vi "D2SParser - Public - Function - Parse File.vi"(8 "error in (no error)":errorcluster, 11 "DS2 File":path) -> (0 "error out":errorcluster, 3 "D2Character":refnum<class "D2Character.lvclass">)   [LabVIEW 2015, in "D2SParser.lvclass"]
uses:
  D2SParser.lvclass
  D2Character/D2Character.lvclass
  D2SParser.lvclass/D2SParser.ctl
  D2SParser - Public - Accessors - Get D2 Character.vi
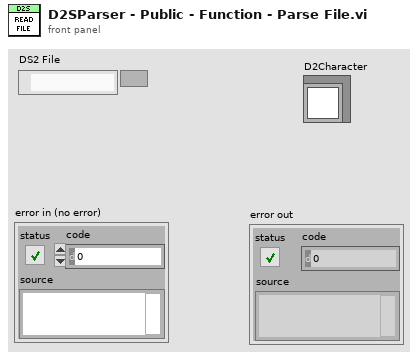
[diagram p1: front panel]
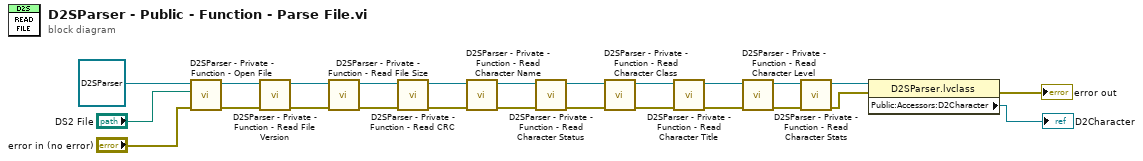
[diagram p0: block diagram]
diagram:
  n1 = call "D2SParser - Private - Function - Open File.vi"("error in (no error)"="error in (no error)", "Path"="DS2 File", "D2SParser in"=refnum<class "D2SParser.lvclass"> refnum) -> ("error out"=w15:errorcluster, "D2SParser out"=w22:refnum<class "D2SParser.lvclass">)  [unwired: 7 in]
  n2 = call "D2SParser - Private - Function - Read File Version.vi"("error in (no error)"=w15, "D2SParser in"=w22) -> ("error out"=w14:errorcluster, "D2SParser out"=w1:refnum<class "D2SParser.lvclass">)  [unwired: 8 in]
  n3 = call "D2SParser - Private - Function - Read File Size.vi"("error in (no error)"=w14, "D2SParser in"=w1) -> ("error out"=w13:errorcluster, "D2SParser out"=w21:refnum<class "D2SParser.lvclass">)  [unwired: 8 in]
  n4 = call "D2SParser - Private - Function - Read CRC.vi"("error in (no error)"=w13, "D2SParser in"=w21) -> ("error out"=w12:errorcluster, "D2SParser out"=w20:refnum<class "D2SParser.lvclass">)  [unwired: 8 in]
  n5 = call "D2SParser - Private - Function - Read Character Name.vi"("error in (no error)"=w12, "D2SParser in"=w20) -> ("error out"=w11:errorcluster, "D2SParser out"=w19:refnum<class "D2SParser.lvclass">)  [unwired: 8 in]
  n6 = call "D2SParser - Private - Function - Read Character Status.vi"("error in (no error)"=w11, "D2SParser in"=w19) -> ("error out"=w10:errorcluster, "D2SParser out"=w18:refnum<class "D2SParser.lvclass">)  [unwired: 8 in]
  n7 = call "D2SParser - Private - Function - Read Character Class.vi"("error in (no error)"=w10, "D2SParser in"=w18) -> ("error out"=w9:errorcluster, "D2SParser out"=w17:refnum<class "D2SParser.lvclass">)  [unwired: 8 in]
  n8 = call "D2SParser - Private - Function - Read Character Title.vi"("error in (no error)"=w9, "D2SParser in"=w17) -> ("error out"=w8:errorcluster, "D2SParser out"=w16:refnum<class "D2SParser.lvclass">)  [unwired: 8 in]
  n9 = call "D2SParser - Private - Function - Read Character Level.vi"("error in (no error)"=w8, "D2SParser in"=w16) -> ("error out"=w4:errorcluster, "D2SParser out"=w5:refnum<class "D2SParser.lvclass">)  [unwired: 8 in]
  n10 = call "D2SParser - Private - Function - Read Character Stats.vi"("error in (no error)"=w4, "D2SParser in"=w5) -> ("error out"=w2:errorcluster, "D2SParser out"=w3:refnum<class "D2SParser.lvclass">)  [unwired: 8 in]
  n11 = property class="D2SParser.lvclass"(reference=w3, error in=w2) -> (error out=→"error out":errorcluster, "Public:Accessors:D2Character"=→"D2Character":refnum<class "D2Character.lvclass">)  [unwired: 1 out]
